vi "Conn New.vi"(4 "error in (no error)":errorcluster, 5 "mode (create new)":T1(ring), 6 "initial data":T2, 7 "object name (unnamed)":string) -> (0 "error out":errorcluster, 1 "status":enum16{"error", "new object", "existing object"}(ring), 3 "connection reference":T3)   [LabVIEW 2013, in "NI_Database_API_64.lvlib"]
doc: "Looks up an existing <B>Connection</B> object matching <B>object name</B> or creates a new Connection object and returns a refnum you can use when calling other Connection methods.\n\n<B>mode</B> specifies whether you want to <B>create</B> a new object or <B>lookup</B> an existing object.\n\n<B>status</B> returns whether a new or an existing object reference is returned.\n\nObjects created with this VI should be destroyed using the <B>Connection Delete</B> VI."
uses:
  NI_Database_API_64.lvlib
  Conn ObjectReference.ctl
  Conn DataMembers.ctl
  <vilib>/Utility/_goopsup.llb/GOOP Object Repository Method.ctl
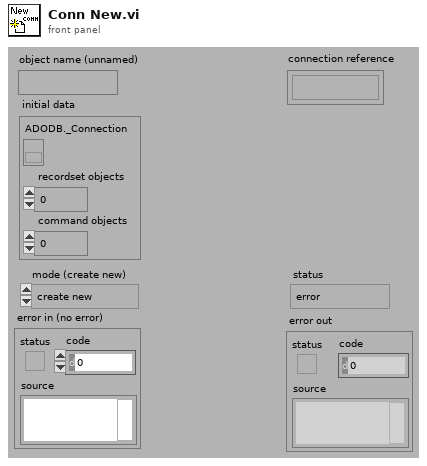
[diagram p1: front panel]
types:
  T1 = enum16{"create new", "lookup existing", "lookup or create"}
  T2 = typedef "NI_Database_API_64.lvlib/Conn DataMembers.ctl" = cluster{"ADODB._Connection":refnum<k7>, "recordset objects":i32, "command objects":i32}
  T3 = typedef "NI_Database_API_64.lvlib/Conn ObjectReference.ctl" = refnum<k1>
  T4 = typedef "GOOP Object Repository Method.ctl" = enum16{"Create", "GetCopy", "GetModify", "Set", "Destroy", "Create Static", "Get All Refs", "Reset", "Get Statistics"}
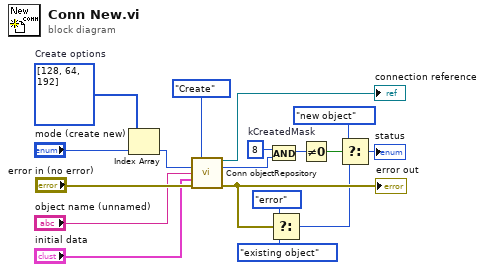
[diagram p0: block diagram]
diagram:
  w9 = i32[] [128, 64, 192]  # Create options
  w12 = 8  # kCreatedMask
  n1 = Index Array(array=w9, index="mode (create new)") -> (element=w8:i32)
  n2 = call "Conn objectRepository.vi"("method"=GOOP_Object_Repository_Method."Create", "flags in"=w8, "name in"="object name (unnamed)", "classDataIn"="initial data", "error in (no error)"="error in (no error)") -> ("connection reference out"=→"connection reference":T3, "flags out"=w11:i32, "error out"=w18:errorcluster)  [unwired: 4 in, 4 out]
  "error out" <- w18
  n3 = And(x=w12, y=w11) -> (x .and. y?=w7:i32)
  n4 = Select(t=enum16{"error", "new object", "existing object"}."error" ("status"), s=w18, f=enum16{"error", "new object", "existing object"}."existing object" ("status")) -> (s? t:f=w2:enum16{"error", "new object", "existing object"})
  n5 = Not Equal To 0?(x=w7) -> (x != 0?=w6:bool)
  n6 = Select(t=enum16{"error", "new object", "existing object"}."new object" ("status"), s=w6, f=w2) -> (s? t:f=→"status":enum16{"error", "new object", "existing object"})
